vi "PIDController_Pack_Tuning.vi"(4 "MinimumIntegral":dbl=-9.9e+30, 6 "MaximumIntegral":dbl=9.9e+30, 7 "Kn":dbl=1.0, 8 "IntegralZone":dbl=9.9e+30, 9 "Kd":dbl, 10 "Ki":dbl, 11 "Kp":dbl) -> (3 "PID Tuning":T1={"Kp"=0.0, "Ki"=0.0, "Kd"=0.0, "MaximumIntegral"=9.9e+30, "MinimumIntegral"=-9.9e+30, "IntegralZone"=9.9e+30})   [LabVIEW 2019, in "Trajectory_Library.lvlib"]
doc: "Convience function to pack individual tuning parameter values into a cluster to pas to the PID controller\n\nInputs:\n - Kn -- Optional normalizing constants. When present, the other constants are multiplied by this constant. Set this equal to the maximum controller output divided by the corresponding maximum process value that corresponds to the maximum controller output. Using this can help simlify tuning.\n - Kp -- Proportional gain constant. The error is multiplied by this value. (Default = 0.0)\n - Ki -- Integral gain constant. The integral of the error is multiplied by this value. (Default = 0.0)\n - Kd -- Derivative gain constant The derivative of the error is multipled by this value. (Default = 0.0)\n - Maximum Integral -- The integral component of the output is not allowed to exceed this value This limits the travel of the integral This is in units of the output value. ( Default = 9.9E+30 )\n - Minimal Integral -- The integral component of the output is not allowed to be less than this value. This limits the travel of the integral This is in units of the output value. ( Default = -9.9E+30 )\n - IntegralZone - double - Absolute value of error (in process variable units) to allow integration. Specifying this value helps to prevent integral windup when moving from one setpoint to another. (Default = 9.9E+30)\n\nOutput:\n - PID Tuning -- Cluster containing the tuning values."
uses:
  Trajectory_Library.lvlib
  TypeDef/PID_TUNING.ctl
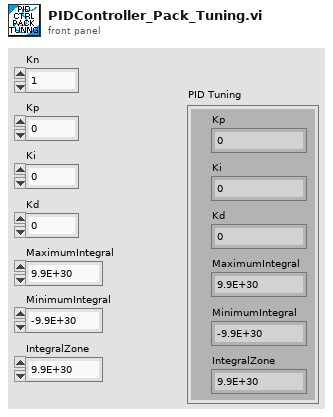
[diagram p1: front panel]
types:
  T1 = typedef "Trajectory_Library.lvlib/PID_TUNING.ctl" = cluster{"Kp":dbl, "Ki":dbl, "Kd":dbl, "MaximumIntegral":dbl, "MinimumIntegral":dbl, "IntegralZone":dbl}
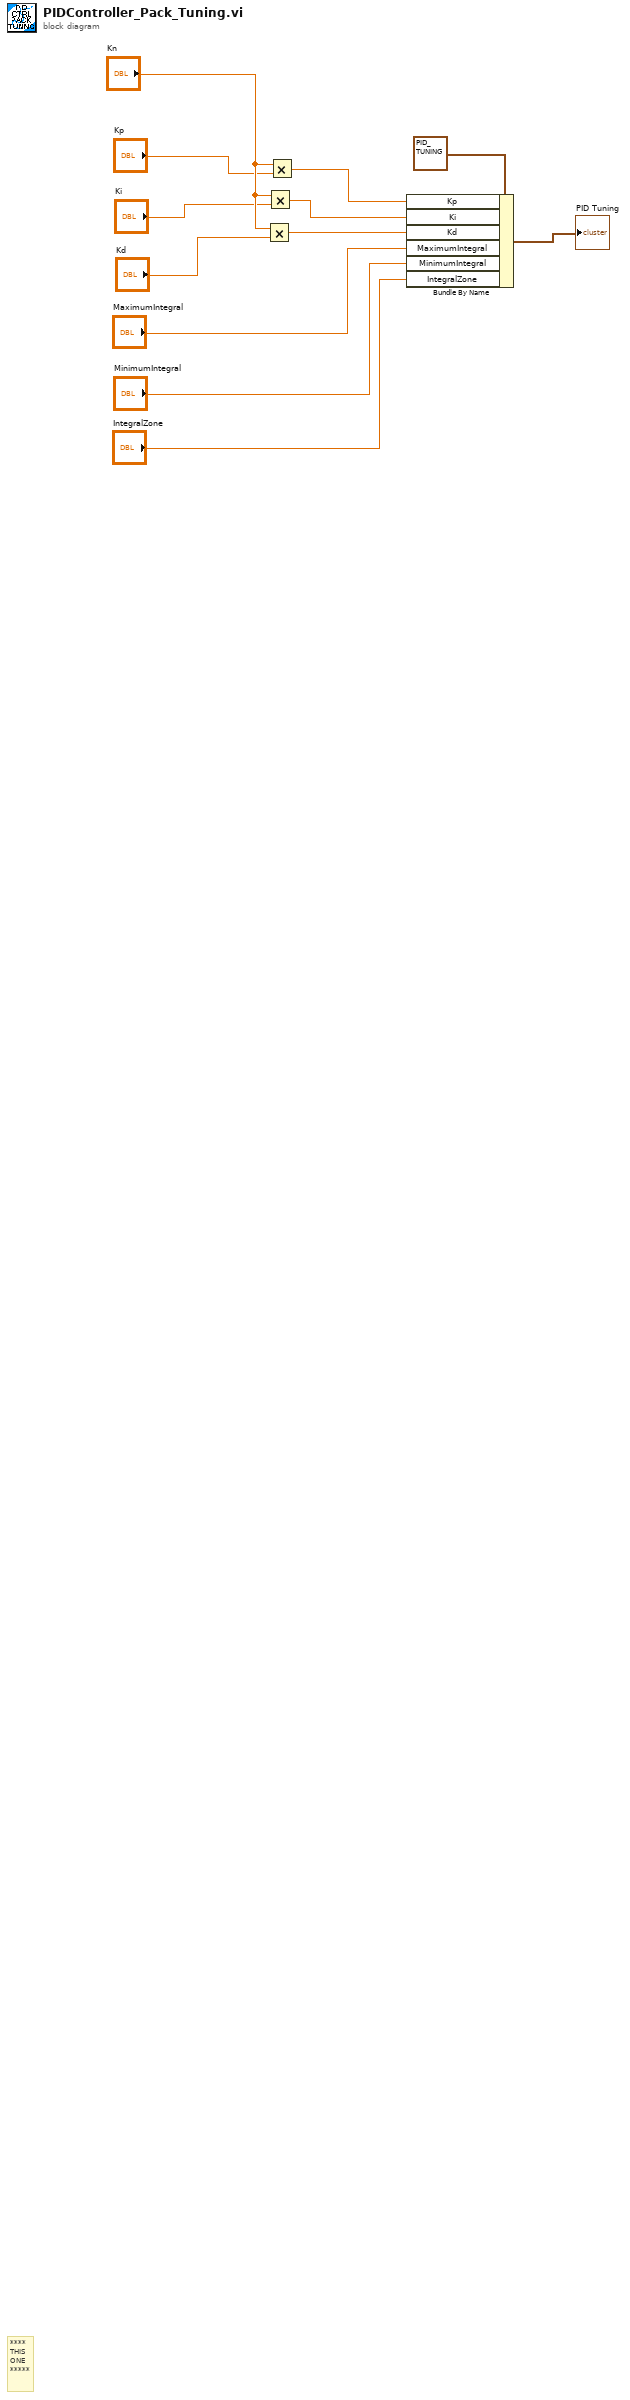
[diagram p0: block diagram]
diagram:
  # "****\nTHIS\nONE\n*****"
  n1 = Multiply(x="Kn", y="Kd") -> (x*y=w8:dbl)
  n2 = Multiply(x="Kn", y="Ki") -> (x*y=w7:dbl)
  n3 = Multiply(x="Kn", y="Kp") -> (x*y=w6:dbl)
  n4 = Bundle By Name(cluster=T1 {"Kp"=0.0, "Ki"=0.0, "Kd"=0.0, "MaximumIntegral"=9.9e+30, "MinimumIntegral"=-9.9e+30, "IntegralZone"=9.9e+30} ("PID Tuning"), "Kp"=w6, "Ki"=w7, "Kd"=w8, "MaximumIntegral"="MaximumIntegral", "MinimumIntegral"="MinimumIntegral", "IntegralZone"="IntegralZone") -> (→"PID Tuning":T1)
